vi "RS485 COM.vi"(11 "Input":T1={"Data"=[0, 0, 0, 0, 0, 0, 0, 0, 0, 0, 0, 0, 0, 0, 0, 0, 0, 0, 0, 0, 0, 0, 0, 0, 0, 0, 0, 0, 0, 0, 0, 0, 0, 0, 0, 0, 0, 0, 0, 0, 0, 0, 0, 0, 0, 0, 0, 0, 0, 0, 0, 0, 0, 0, 0, 0, 0, 0, 0, 0, 0, 0, 0, 0, 0, 0, 0, 0, 0, 0, 0, 0, 0, 0, 0, 0, 0, 0, 0, 0, 0, 0, 0, 0, 0, 0, 0, 0, 0, 0, 0, 0, 0, 0, 0, 0, 0, 0, 0, 0, 0, 0, 0, 0, 0, 0, 0, 0, 0, 0, 0, 0, 0, 0, 0, 0, 0, 0, 0, 0, 0, 0, 0, 0, 0, 0, 0, 0, 0, 0, 0, 0, 0, 0, 0, 0, 0, 0, 0, 0, 0, 0, 0, 0, 0, 0, 0, 0, 0, 0, 0, 0, 0, 0, 0, 0, 0, 0, 0, 0, 0, 0, 0, 0, 0, 0, 0, 0, 0, 0, 0, 0, 0, 0, 0, 0, 0, 0, 0, 0, 0, 0, 0, 0, 0, 0, 0, 0, 0, 0, 0, 0, 0, 0, 0, 0, 0, 0, 0, 0], "NumBytes"=0, "RS485_Cmd"=enum."Read", "Port"=enum."Port 1", "Timeout (ms)"=0, "New"=FALSE}) -> (0 "error IO":errorcluster)   [LabVIEW 2015]
uses:
  <vilib>/eio/EIOMethodNode/EIOMethodNode.xnode
  <vilib>/rvi/eio/common/nirviEmuTemplateMethod_errors.vi
  RS485 In.ctl
  Port.ctl
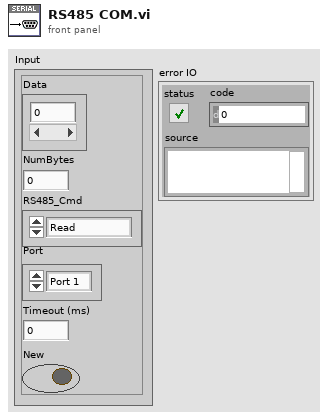
[diagram p1: front panel]
types:
  T1 = typedef "RS485 In.ctl" = cluster{"Data":u8[], "NumBytes":i32, "RS485_Cmd":enum8{"Read", "Write", "Idle"}, "Port":T2, "Timeout (ms)":i32, "New":bool}
  T2 = typedef "Port.ctl" = enum8{"Port 1", "Port 2", "Port 3", "Port 4", "None"}
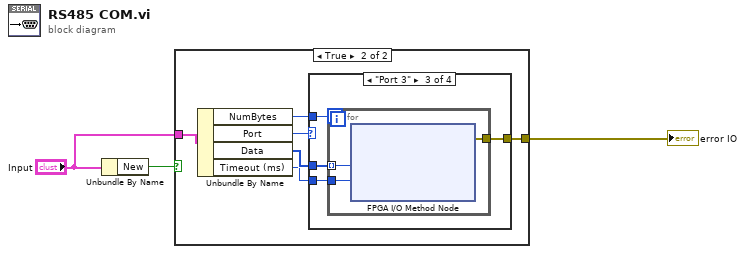
[diagram p0: block diagram]
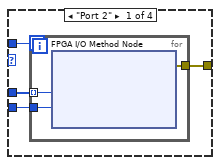
[diagram p3: hidden frame]
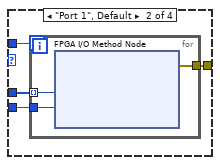
[diagram p4: hidden frame]
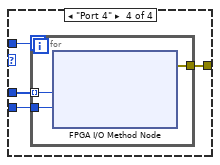
[diagram p5: hidden frame]
diagram:
  n1 = Unbundle By Name("Input") -> ("New"=w3:bool)
  n2 = case shown="True" w3 {
    tunnel: "Input" -> [_ w9]
    tunnel: [_ w5] -> w1
    frame False {
    }
    frame True {
      n3 = Unbundle By Name(w9) -> ("NumBytes"=w8:i32, "Port"=w6:T2, "Data"=w7:u8[], "Timeout (ms)"=w4:i32)
      n4 = case shown="\"Port 3\"" w6 {
        tunnel: w8 -> [w13 w20 w27 w34]
        tunnel: w7 -> [w12 w19 w26 w33]
        tunnel: [w11 w18 w25 w32] -> w5
        tunnel: w4 -> [w10 w17 w24 w31]
        frame "Port 2" {
          n5 = for {
            N: w13 -> [_]
            tunnel: w12 -> [w16] mode=indexing
            tunnel: w10 -> [w15]
            tunnel: [w14] -> w11
            n6 = xnode "FPGA I/O Method Node"("Data"=w16, "Timeout (ms)"=w15) -> ("error out"=w14:errorcluster)  [unwired: 2 in, 2 out]
          }
        }
        frame "Port 1", Default {
          n7 = for {
            N: w20 -> [_]
            tunnel: w19 -> [w23] mode=indexing
            tunnel: w17 -> [w22]
            tunnel: [w21] -> w18
            n8 = xnode "FPGA I/O Method Node"("Data"=w23, "Timeout (ms)"=w22) -> ("error out"=w21:errorcluster)  [unwired: 2 in, 2 out]
          }
        }
        frame "Port 3" {
          n9 = for {
            N: w27 -> [_]
            tunnel: w26 -> [w30] mode=indexing
            tunnel: w24 -> [w29]
            tunnel: [w28] -> w25
            n10 = xnode "FPGA I/O Method Node"("Data"=w30, "Timeout (ms)"=w29) -> ("error out"=w28:errorcluster)  [unwired: 2 in, 2 out]
          }
        }
        frame "Port 4" {
          n11 = for {
            N: w34 -> [_]
            tunnel: w33 -> [w37] mode=indexing
            tunnel: w31 -> [w36]
            tunnel: [w35] -> w32
            n12 = xnode "FPGA I/O Method Node"("Data"=w37, "Timeout (ms)"=w36) -> ("error out"=w35:errorcluster)  [unwired: 2 in, 2 out]
          }
        }
      }
    }
  }
  "error IO" <- w1
